vi "Actor Core.vi"(8 "error in":errorcluster, 11 "Nested in":refnum<class "MDI Panel Actor.lvclass">) -> (0 "error out":errorcluster, 3 "Actor out":refnum<class "Actor.lvclass">)   [LabVIEW 2018, in "MDI Panel Actor.lvlib" / "MDI Panel Actor.lvclass"]
doc: "(<B>Filename</B>: Actor Framework.lvlib:Actor.lvclass:Actor Core.vi)\n\nReceives messages to the actor, reacts to them, and initiates any error handling that may shut the actor down.\n\nDescendant classes may override this VI to append parallel tasks for the actor to complete while it handles messages. Overrides use the Call Parent Method node."
uses:
  MDI Panel Actor.lvclass
  D:/Program Files (x86)/National Instruments/LabVIEW 2018/vi.lib/MGI/Panel Manager/Panel Actor/Panel Actor/Panel Actor.lvclass
  <vilib>/ActorFramework/Actor/Actor.lvclass
  System.Windows.Forms
  <vilib>/ActorFramework/Message Enqueuer/Message Enqueuer.lvclass
  MDI Panel Actor.lvclass/MDI Panel Actor.ctl
  <vilib>/ActorFramework/Message Enqueuer/Message Enqueuer.lvclass/Message Enqueuer.ctl
  Chart Actor/Chart Actor.lvclass
  <vilib>/MGI/Panel Manager/Panel/Window Position/Reference Position/Alignment.ctl
  <vilib>/MGI/Panel Manager/Panel/Window Position/Reference Position/Horizontal Alignment.ctl
  <vilib>/MGI/Panel Manager/Panel/Window Position/Reference Position/Vertical Alignment.ctl
  <vilib>/MGI/Panel Manager/Panel/Window Position/Reference Position/Size/Reference Size/Reference Size.lvclass/Reference Size.ctl
  <vilib>/MGI/Panel Manager/Panel/Window Position/Reference Position/Size/Reference Size/Reference Size.vi
  <vilib>/ActorFramework/Message Enqueuer/Enqueue.vi
  <vilib>/ActorFramework/Stop Msg/Stop Msg.lvclass
  D:/Program Files (x86)/National Instruments/LabVIEW 2018/vi.lib/ActorFramework/Message/Message.lvclass
  <vilib>/MGI/Panel Manager - .NET Panels/MDI/MDI Panel/MDI Panel.lvclass
  D:/Program Files (x86)/National Instruments/LabVIEW 2018/vi.lib/MGI/Panel Manager/Panel/Panel/Panel.lvclass
  <vilib>/MGI/Panel Manager/Panel/Panel/Window/Window.lvclass
  <vilib>/ActorFramework/Message Priority Queue/Priority Enqueue.vi
  <vilib>/MGI/Panel Manager - .NET Panels/MDI/MDI Panel/MDI Panel_Sized Window.vi
  <vilib>/MGI/Panel Manager/Panel/Panel/Window/Window.vi
  <vilib>/MGI/Panel Manager - .NET Panels/MDI/MDI Panel/MDI Panel_Maximized Window.vi
  <vilib>/MGI/Panel Manager/Panel/Window Position/Reference Position/Size/Reference Size/Reference Size.lvclass
  <vilib>/MGI/Panel Manager/Panel Actor/Panel Actor/Panel Actor.lvclass
  <vilib>/MGI/Panel Manager - .NET Panels/MDI/MDI Container/MDI Container.lvclass
  <vilib>/MGI/Panel Manager/Panel Actor/Panel Actor Messages/Change Panel Msg/Change Panel Msg.lvclass
  <vilib>/MGI/Panel Manager/Panel/Panel.lvlib
  <vilib>/MGI/Panel Manager/Panel/Window Position/Reference Position/Reference Position.lvclass
panel:
  in  "Panel":refnum<k24>(container)
  in  "Lock":bool
  in  "unlock":bool
  in  "New Panel":bool
  in  "Cascade":bool
  in  "Tile V":bool
  in  "Tile H":bool
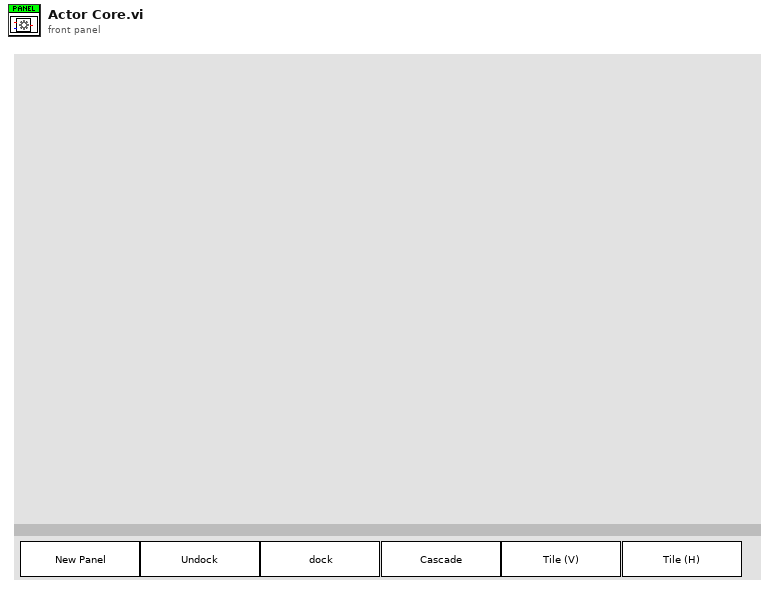
[diagram p1: front panel]
types:
  T1 = cluster{"事件注册引用句柄":refnum<event-registration>, "Pnl Actor":refnum<event-registration>}
  T2 = typedef "Panel.lvlib/Reference Position.lvclass/Alignment.ctl" = cluster{"Horizontal":T3, "Vertical":T4}
  T3 = typedef "Panel.lvlib/Reference Position.lvclass/Horizontal Alignment.ctl" = enum16{"Left", "Center", "Right"}
  T4 = typedef "Panel.lvlib/Reference Position.lvclass/Vertical Alignment.ctl" = enum16{"Top", "Center", "Bottom"}
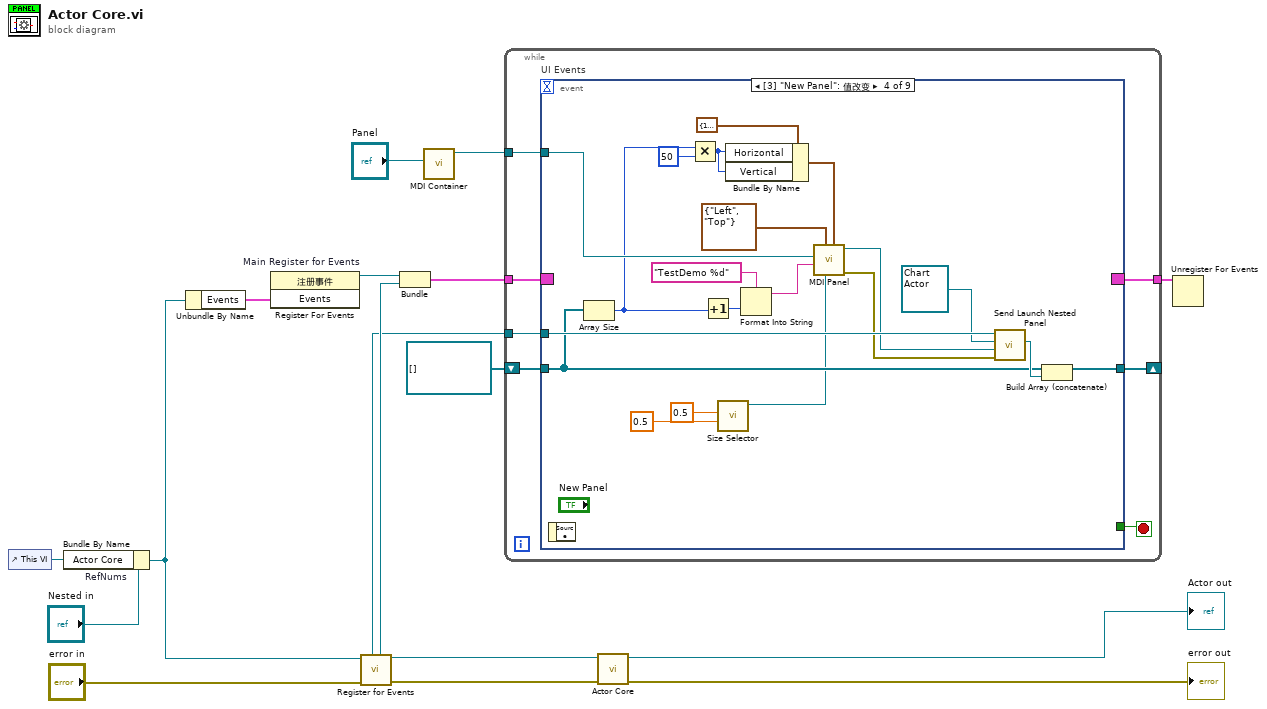
[diagram p0: block diagram]
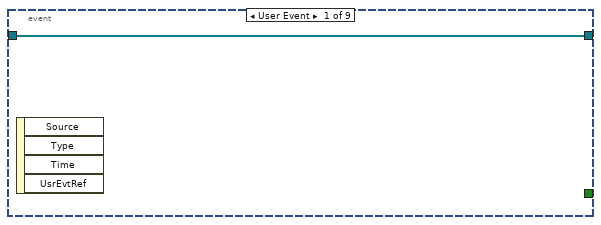
[diagram p2: hidden frame]
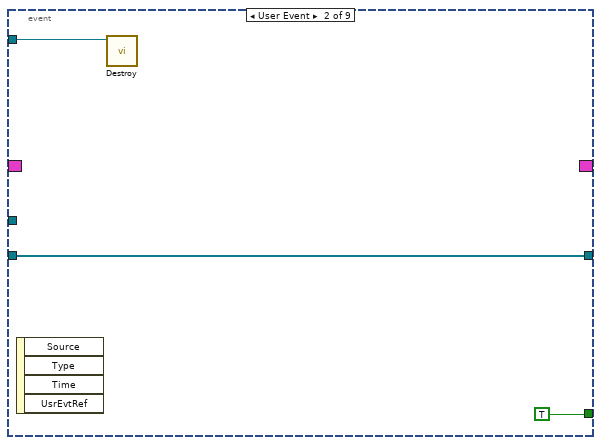
[diagram p3: hidden frame]
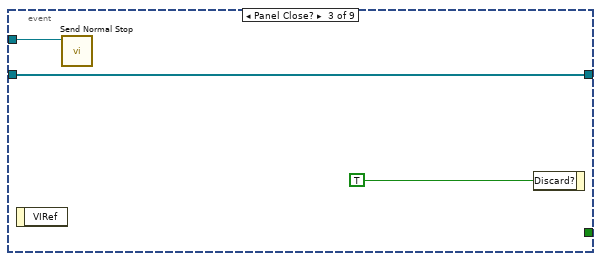
[diagram p4: hidden frame]
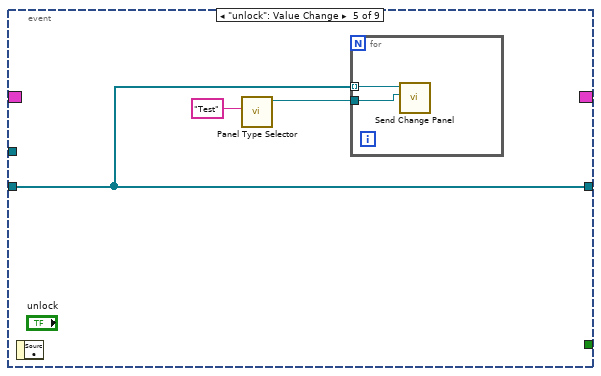
[diagram p5: hidden frame]
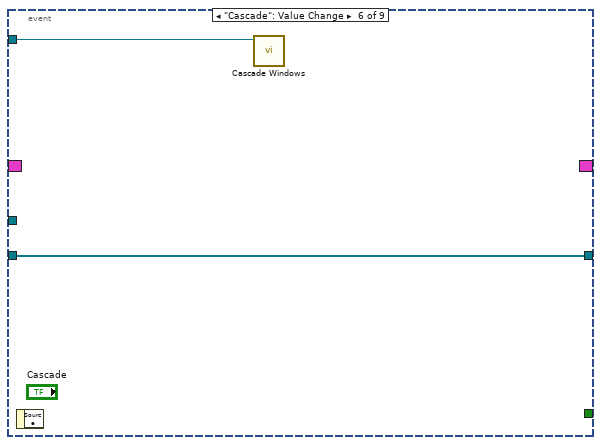
[diagram p6: hidden frame]
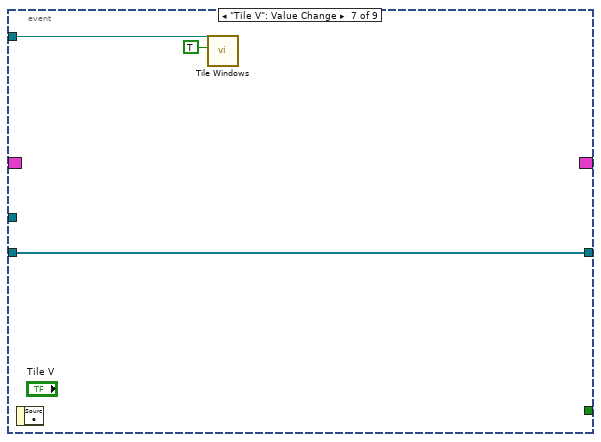
[diagram p7: hidden frame]
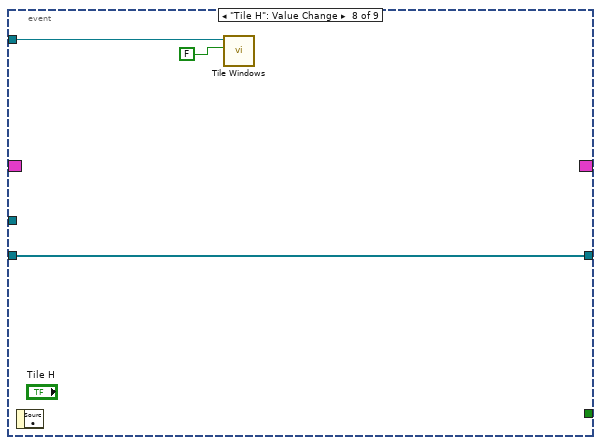
[diagram p8: hidden frame]
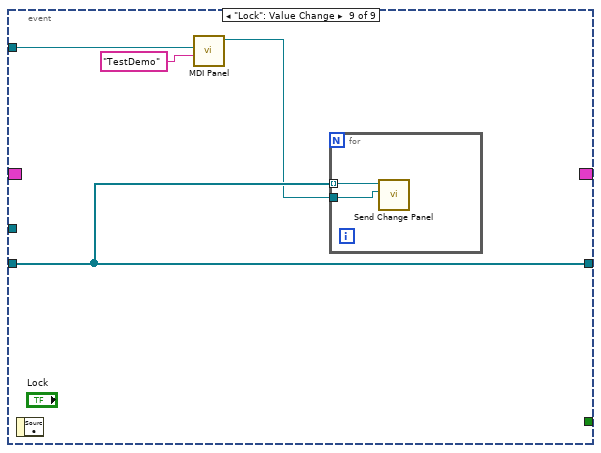
[diagram p9: hidden frame]
diagram:
  n1 = control-ref of="This VI"() -> (w12:refnum<vi>)
  n2 = Bundle By Name "RefNums"(cluster="Nested in", "Actor Core"=w12) -> (w5:refnum<class "MDI Panel Actor.lvclass">)
  n3 = Unbundle By Name(w5) -> ("Events"=w15:cluster{"Stop":refnum<user-event>})
  n4 = register-events "Main Register for Events"(w15) -> (reference out=w9:refnum<event-registration>)  [unwired: 2 in, 1 out]
  n5 = call <vilib>:"Register for Events.vi"("Error In"="error in", "Panel Actor in"=w5) -> ("Error Out"=w10:errorcluster, "Panel Actor out"=w11:refnum<class "MDI Panel Actor.lvclass">, "Pnl Actor"=w7:refnum<event-registration>, "Self Enqueuer"=w6:refnum<class "Message Enqueuer.lvclass">)  [unwired: 6 in]
  n6 = Bundle("事件注册引用句柄"=w9, "Pnl Actor"=w7) -> (w8:T1)  [unwired: 1 in]
  n7 = call <vilib>:"MDI Container.vi"("Panel"="Panel") -> ("Container out"=w2:refnum<class "MDI Container.lvclass">)  [unwired: 9 in, 1 out]
  n8 = while {
    tunnel: w8 -> [w24]
    tunnel: [w22] -> w14
    tunnel: w6 -> [w21]
    tunnel: w2 -> [w20]
    shift-right: [w19] -> _
    shift-left: refnum<class "Message Enqueuer.lvclass">[] [] -> [w18]
    stop <- w23 stop-if-true
    n9 = event "UI Events" shown="[3] \"New Panel\": 值改变" {
      selector: w24 -> [_ _ _ _ _ _ _ _ _]
      dyn-events: [_ _ _ _ _ _ _ _ _] -> w22
      timeout: _ -> [_ _ _ _ _ _ _ _ _]
      tunnel: [_ TRUE _ _ _ _ _ _ _] -> w23
      tunnel: w21 -> [_ _ w30 w51 _ _ _ _ _]
      tunnel: w20 -> [_ w26 _ w47 _ w58 w61 w63 w67]
      tunnel: [w25 w27 w29 w48 w54 w57 w59 w62 w68] -> w19
      tunnel: w18 -> [w25 w27 w29 w45 w54 w57 w59 w62 w68]
      event User Event {
        n10 = event-data() -> ()  [unwired: 1 in, 4 out]
      }
      event User Event {
        n11 = event-data() -> ()  [unwired: 1 in, 4 out]
        n12 = call <vilib>:"Destroy.vi"("Container in"=w26) -> ()  [unwired: 10 in, 1 out]
      }
      event Panel Close? {
        n13 = event-data() -> ()  [unwired: 1 in, 1 out]
        n14 = call <vilib>:"Send Normal Stop.vi"("Message Enqueuer"=w30) -> ()  [unwired: 10 in, 1 out]
        n15 = event-data("Discard?"=TRUE) -> ()  [unwired: 1 in, 1 out]
      }
      event "New Panel": Value Change {
        n16 = event-data() -> ()  [unwired: 1 in, 1 out]
        n17 = Array Size(array=w45) -> (size(s)=w36:i32)
        n18 = Multiply(x=w36, y=50) -> (x*y=w32:i32)
        n19 = Increment(x=w36) -> (x+1=w44:i32)
        n20 = call-poly <vilib>:"Size Selector.vi"("Height Scale"=0.5, "Width Scale"=0.5) -> ("Static Out"=w41:refnum<class "Reference Size.lvclass">)  [unwired: 8 in, 1 out]
        n21 = Bundle By Name(cluster=cluster{"Horizontal":i16, "Vertical":i16} {"Horizontal"=100, "Vertical"=0} ("Offset"), "Horizontal"=w32, "Vertical"=w32) -> (w33:cluster{"Horizontal":i16, "Vertical":i16})
        n22 = Format Into String(format string="TestDemo %d" ("Title"), w44) -> (resulting string=w42:string)  [unwired: 2 in, 1 out]
        n23 = call-poly <vilib>:"MDI Panel.vi"("Offset"=w33, "Size"=w41, "Alignment"=T2 {"Horizontal"=enum."Left", "Vertical"=enum."Top"}, "Title"=w42, "MDI Container"=w47) -> ("error out"=w38:errorcluster, "MDI Panel out"=w46:refnum<class "MDI Panel.lvclass">)  [unwired: 5 in]
        n24 = call <vilib>:"Send Launch Nested Panel.vi"("Error In"=w38, "Panel"=w46, "Nested Panel Actor"=refnum<class "Chart Actor.lvclass"> refnum ("Chart Actor.lvlib:Chart Actor.lvclass"), "Self Enqueuer in"=w51) -> ("Nested Actor's Enqueuer"=w49:refnum<class "Message Enqueuer.lvclass">)  [unwired: 6 in, 1 out]
        n25 = Build Array (concatenate)(w45, w49) -> (w48:refnum<class "Message Enqueuer.lvclass">[])
      }
      event "unlock": Value Change {
        n26 = event-data() -> ()  [unwired: 1 in, 1 out]
        n27 = call-poly <vilib>:"Panel Type Selector.vi"("Default Title"="Test") -> ("Window out"=w53:refnum<class "Window.lvclass">)  [unwired: 9 in, 1 out]
        n28 = for {
          tunnel: w54 -> [w56] mode=indexing
          tunnel: w53 -> [w55]
          n29 = call <vilib>:"Send Change Panel.vi"("New Panel"=w55, "Message Enqueuer in"=w56) -> ()  [unwired: 8 in, 2 out]
        }
      }
      event "Cascade": Value Change {
        n30 = event-data() -> ()  [unwired: 1 in, 1 out]
        n31 = call <vilib>:"Cascade Windows.vi"("Container in"=w58) -> ()  [unwired: 10 in, 1 out]
      }
      event "Tile V": Value Change {
        n32 = event-data() -> ()  [unwired: 1 in, 1 out]
        n33 = call <vilib>:"Tile Windows.vi"("Vertical?"=TRUE, "Container in"=w61) -> ()  [unwired: 9 in, 1 out]
      }
      event "Tile H": Value Change {
        n34 = event-data() -> ()  [unwired: 1 in, 1 out]
        n35 = call <vilib>:"Tile Windows.vi"("Vertical?"=FALSE, "Container in"=w63) -> ()  [unwired: 9 in, 1 out]
      }
      event "Lock": Value Change {
        n36 = event-data() -> ()  [unwired: 1 in, 1 out]
        n37 = call-poly <vilib>:"MDI Panel.vi"("Title"="TestDemo", "MDI Container"=w67) -> ("MDI Panel out"=w66:refnum<class "MDI Panel.lvclass">)  [unwired: 8 in, 1 out]
        n38 = for {
          tunnel: w68 -> [w70] mode=indexing
          tunnel: w66 -> [w69]
          n39 = call <vilib>:"Send Change Panel.vi"("New Panel"=w69, "Message Enqueuer in"=w70) -> ()  [unwired: 8 in, 2 out]
        }
      }
    }
  }
  n40 = call-parent "Actor Core.vi"("error in"=w10, "Panel Actor in"=w11) -> ("error out"=→"error out":errorcluster, "Actor out"=→"Actor out":refnum<class "Actor.lvclass">)  [unwired: 8 in]
  n41 = Unregister For Events(event registration refnum=w14) -> ()  [unwired: 1 in, 1 out]
